vi "Add Tool Offset.vi"(11 "XYZTheta":dbl[](array[numeric])) -> (3 "Array":dbl[](array[numeric]))   [LabVIEW 2020, in "Pick and Place.lvclass"]
uses:
  Pick and Place.lvclass
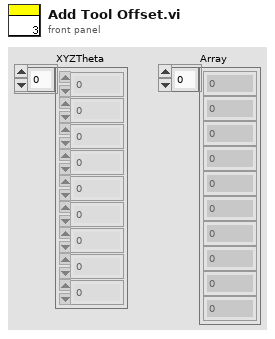
[diagram p1: front panel]
types:
  T1 = typedef "File Paths.ctl" = cluster{"Glue Pattern Folder":path, "Carrier Tray Folder":path, "Pick Up Tool Fixture Folder":path, "Components Folder":path, "Bellows Tool Offset.txt":path, "Pick Up Tool Offset.txt":path, "Dispense Tip Offset.txt":path, "Log Files":path, "Gantry Assembly Map.txt":path, "Syringe and offset map.txt":path}
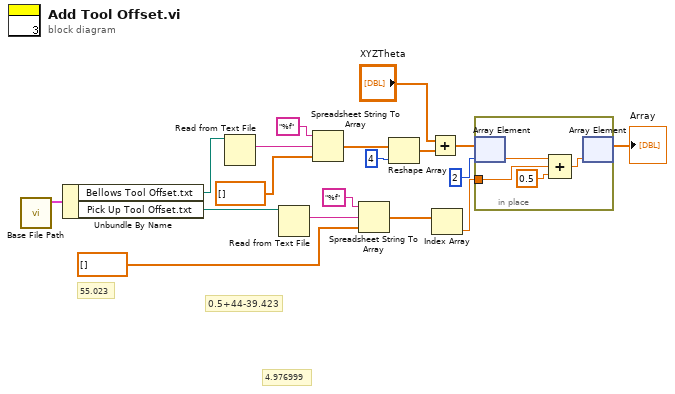
[diagram p0: block diagram]
diagram:
  # "55.023"
  # "4.976999"
  # "0.5+44-39.423"
  n1 = call "Base File Path.vi"() -> ("Paths Out"=w11:T1)  [unwired: 11 in]
  n2 = Unbundle By Name(w11) -> ("Bellows Tool Offset.txt"=w12:path, "Pick Up Tool Offset.txt"=w4:path)
  n3 = Read from Text File(file (use dialog)=w12) -> (text=w13:string)  [unwired: 3 in, 3 out]
  n4 = Read from Text File(file (use dialog)=w4) -> (text=w7:string)  [unwired: 3 in, 3 out]
  n5 = Spreadsheet String To Array(format string="%f", spreadsheet string=w13, array type (2D Dbl)=dbl[] []) -> (array=w16:dbl[])  [unwired: 1 in]
  n6 = Spreadsheet String To Array(format string="%f", spreadsheet string=w7, array type (2D Dbl)=dbl[] []) -> (array=w3:dbl[])  [unwired: 1 in]
  n7 = Reshape Array(w16, 4 ("dimension size")) -> (w18:dbl[])
  n8 = Add(x="XYZTheta", y=w18) -> (x+y=w10:dbl[])
  n9 = Index Array(array=w3) -> (element=w2:dbl)  [unwired: 1 in]
  n10 = in-place {
    in-place-border: w2 -> [w21]
    n11 = in-place-array #1(w10, 2) -> (w22:dbl)
    n12 = Compound Arithmetic op=ADD(w22, w21, 0.5 ("x")) -> (w20:dbl)
    n13 = in-place-array #1(w20) -> (→"Array":dbl[])  [unwired: 1 out]
  }
